vi "Measurement Logic.vi"() -> ()   [LabVIEW 2021, in "DAQmxMeasurement1.lvlib"]
uses:
  DAQmxMeasurement1.lvlib
  <vilib>/Plug-In SDKs/Measurements/Measure Call Context/Measure Call Context.lvclass
  Measurement Configuration.ctl
  Measurement Results.ctl
  <vilib>/Plug-In SDKs/Clients/Session Management V1/Session Reservation/Initialize and Close Session Behavior.ctl
  <vilib>/Plug-In SDKs/Measurements/Measure Call Context/Reserve Sessions - 1Pin.vi
  Sessions/niDAQmx/Initialize Tasks - 1Task.vi
  Sessions/niDAQmx/Get Connections - 1Pin 1Conn.vi
  Sessions/niDAQmx/Session Management niDAQmx.lvlib
  <vilib>/Plug-In SDKs/Clients/Session Management V1/Session Reservation/Session Reservation.lvclass
panel:
  out "measurement results":T1
  in  "measurement configuration":T2={"pin_name"="Lorem ipsum dolor sit"}
  out "measure call context out":refnum<class "Measure Call Context.lvclass">
  in  "measure call context in":refnum<class "Measure Call Context.lvclass">
  out "error out":errorcluster
  in  "error in":errorcluster
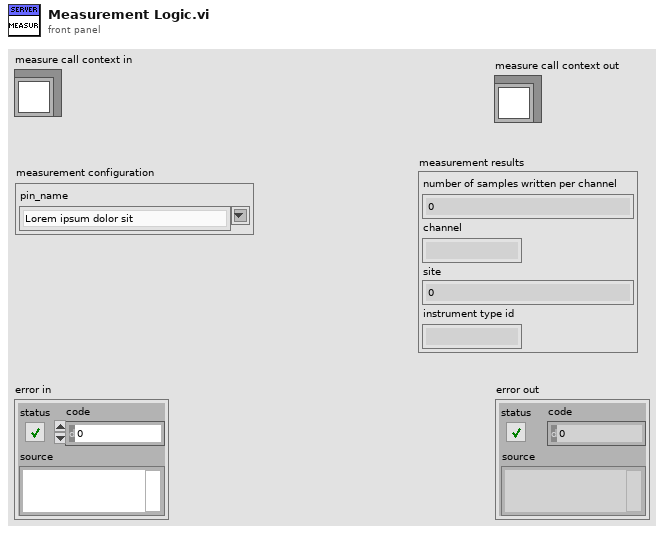
[diagram p1: front panel]
types:
  T1 = typedef "DAQmxMeasurement1.lvlib/Measurement Results.ctl" = cluster{"number of samples written per channel":u32, "channel":string, "site":i32, "instrument type id":string}
  T2 = typedef "DAQmxMeasurement1.lvlib/Measurement Configuration.ctl" = cluster{"pin_name":string}
  T3 = typedef "NI Session Management V1 Client.lvlib/Session Reservation.lvclass/Initialize and Close Session Behavior.ctl" = enum16{"Auto", "Initialize and Close", "Attach and Detach", "Initialize and Detach", "Attach and Close"}
  T4 = typedef "Session Management niDAQmx.lvlib/Connection with Session.ctl" = cluster{"connection":T5, "session":refnum<class "Session Factory.lvclass">}
  T5 = typedef "NI Session Management V1 Client.lvlib/Session Reservation.lvclass/Connection.ctl" = cluster{"pin or relay name":string, "site":i32, "instrument type id":string, "channel":string}
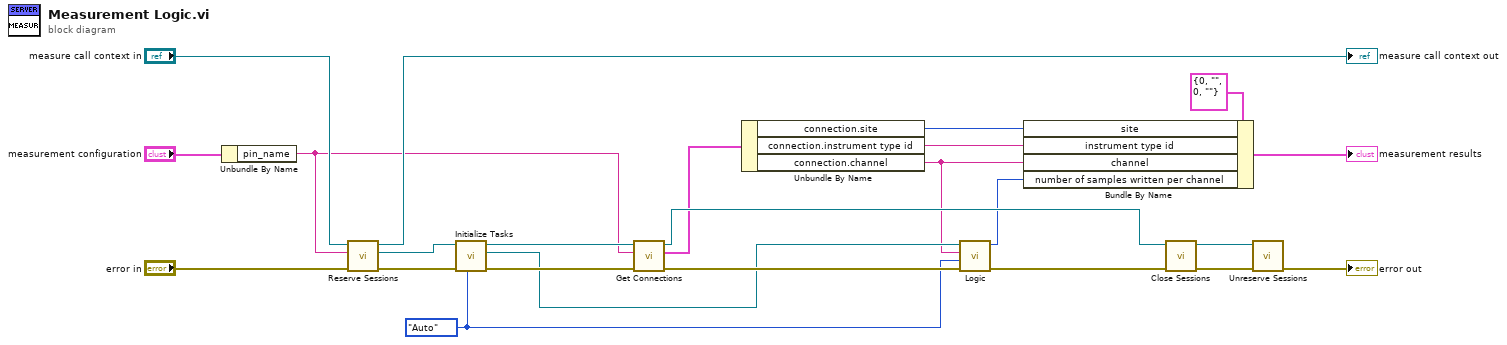
[diagram p0: block diagram]
diagram:
  w3 = Initialize_and_Close_Session_Behavior."Auto" ("initialize and close session behavior")
  n1 = Unbundle By Name("measurement configuration") -> ("pin_name"=w9:string)
  n2 = call-poly <vilib>:"Reserve Sessions.vi"("error in"="error in", "pin or relay name"=w9, "measurement context in"="measure call context in") -> ("error out"=w20:errorcluster, "session reservation out"=w17:refnum<class "Session Reservation.lvclass">, "measurement context out"=→"measure call context out":refnum<class "Measure Call Context.lvclass">)  [unwired: 6 in]
  n3 = call-poly "Initialize Tasks.vi"("initialize and close session behavior"=w3, "error in"=w20, "session reservation in"=w17) -> ("error out"=w13:errorcluster, "task"=w4:refnum<class "Session Factory.lvclass">, "session reservation out"=w12:refnum<class "Session Reservation.lvclass">)  [unwired: 5 in, 1 out]
  n4 = call-poly "Get Connections.vi"("error in"=w13, "pin or relay name"=w9, "session reservation in"=w12) -> ("error out"=w5:errorcluster, "connection"=w10:T4, "session reservation out"=w11:refnum<class "Session Reservation.lvclass">)  [unwired: 6 in]
  n5 = Unbundle By Name(w10) -> ("connection.site"=w8:i32, "connection.instrument type id"=w7:string, "connection.channel"=w1:string)
  n6 = call "Logic.vi"("error in (no error)"=w5, "initialize and close session behavior"=w3, "channel list"=w1, "Session Factory in"=w4) -> ("error out"=w6:errorcluster, "number of samples written per channel"=w2:u32)  [unwired: 6 in]
  n7 = Bundle By Name(cluster=T1 {"number of samples written per channel"=0, "channel"="", "site"=0, "instrument type id"=""} ("Measurement Results"), "site"=w8, "instrument type id"=w7, "channel"=w1, "number of samples written per channel"=w2) -> (→"measurement results":T1)
  n8 = call <vilib>:"Close Sessions.vi"("error in"=w6, "session reservation in"=w11) -> ("error out"=w16:errorcluster, "session reservation out"=w14:refnum<class "Session Reservation.lvclass">)  [unwired: 8 in]
  n9 = call <vilib>:"Unreserve Sessions.vi"("error in"=w16, "session reservation in"=w14) -> ("error out"=→"error out":errorcluster)  [unwired: 9 in]
